vi "Main.vi"() -> ()   [LabVIEW 2013] (continued)
                n1844 = call "Msgbox - Message Handler.vi"("Short Description (When DB Not Available)"=w2943, "Description (When DB Not Available)"=w2949, "Post-Description"=w2946, "<.?....> Message Code"=w2944) -> ("MHandler Error"=w2950:errorcluster)  [unwired: 5 in, 2 out]
                n1845 = local write "MHandler"(w2950) -> ()
              }
            }
          }
          frame True {
            # "Must assume that ALL Captions are in Unicode IF IsUnicode is TRUE"
            # "Empty String in Mandatory Field"
            n1846 = call "Msgbox - Message Handler.vi"("Short Description (When DB Not Available)"="Part Details Incomplete" ("string"), "Description (When DB Not Available)"=" must be entered." ("message"), "Pre-Description"=w2960, "<.?....> Message Code"="<E 203>") -> ("MHandler Error"=w2964:errorcluster)  [unwired: 5 in, 2 out]
            n1847 = local write "MHandler"(w2964) -> ()
          }
        }
      }
      event "Part Details": Value Change {
        # "MCListbox Columns order# must match Item Details order#"
        # "USER Clicks on Part Details MCListBox (Also Called by Item No. Value Change}\nUpdate Edit Fields on Top"
        n1848 = event-data() -> ("CtlRef"=w3076:refnum<vi>, "NewVal"=w3070:i32)  [unwired: 1 in, 4 out]
        n1849 = disable-structure shown="Disabled" {
          frame Disabled {
            w3077 = ""
            # "Clear UI"
            n1850 = local write "[Remarks] +[ShortDescription] Debug"(w3077) -> ()
            n1851 = local write "[Remarks] +[ShortDescription]"(w3077) -> ()
          }
          frame Enabled {
          }
        }
        n1852 = property class="MCListbox (strict)"(reference=w3076) -> ("ColHdrString"=w3075:string[], "ItemNames"=w3069:string[][], "Value"=w3073:i32)  [unwired: 1 in, 2 out]
        n1853 = Index Array(array=w3069, index (row)=w3073) -> (element=w3074:string[])  [unwired: 1 in]
        n1854 = case shown="0, Default" w3073 {
          tunnel: w3075 -> [w3117 _]
          tunnel: w3074 -> [w3100 _]
          tunnel: [T30."Enabled" ("Disabled") T30."Disabled and Grayed Out" ("Disabled")] -> w3072
          tunnel: [w3101 T30."Disabled and Grayed Out" ("Disabled")] -> w3071
          tunnel: w3069 -> [_ _]
          frame 0, Default {
            # "Can look at Long Text"
            # "Don't Chnage User"
            # "Exisiting Parts Detail Record"
            n1855 = control-ref of="Item Details"() -> (w3116:refnum<vi>)
            n1856 = control-ref of="Channel Mapping"() -> (w3113:refnum<vi>)
            n1857 = control-ref of="Plot"() -> (w3110:refnum<vi>)
            n1858 = property class="Clust (strict)"(reference=w3116) -> ("Controls[]"=w3115:refnum<vi>[])  [unwired: 1 in, 2 out]
            n1859 = control-ref of="User"() -> ()  [unwired: 1 out]
            n1860 = property class="Clust (strict)"(reference=w3110) -> ("Controls[]"=w3109:refnum<vi>[])  [unwired: 1 in, 2 out]
            n1861 = property class="Clust (strict)"(reference=w3113) -> ("Controls[]"=w3112:refnum<vi>[])  [unwired: 1 in, 2 out]
            n1862 = control-ref of="Notes"() -> (w3114:refnum<vi>)
            n1863 = Build Array (concatenate)(w3115, w3114, w3112, w3109) -> (w3111:refnum<vi>[])
            n1864 = for {
              tunnel: w3111 -> [w3163] mode=indexing
              tunnel: w3117 -> [w3160]
              tunnel: w3100 -> [w3157]
              tunnel: [w3156] -> w3099
              tunnel: [w3156] -> w3107 mode=indexing
              n1865 = property class="Ctl"(reference=w3163) -> (reference out=w3161:refnum<vi>, "Label.Text"=w3159:string, "ClassName"=w3162:string)  [unwired: 1 in, 1 out]
              n1866 = Search 1D Array(1D array=w3160, element=w3159) -> (index of element=w3158:i32)  [unwired: 1 in]
              n1867 = case shown="0, Default" w3158 {
                selector: w3158 -> [w3165 _]
                tunnel: w3157 -> [w3169 _]
                tunnel: w3162 -> [w3168 _]
                tunnel: w3161 -> [w3166 _]
                tunnel: [w3164 _] -> w3156
                frame 0, Default {
                  n1868 = Index Array(array=w3169, index=w3165) -> (element=w3167:string)
                  n1869 = case shown="\"Boolean\"" w3168 {
                    tunnel: w3167 -> [w3172 w3176 w3179]
                    tunnel: w3166 -> [w3171 w3175 w3180]
                    tunnel: [w3170 w3174 w3177] -> w3164
                    frame "Digital" {
                      n1870 = Decimal String To Number(string=w3172) -> (number=w3173:i32)  [unwired: 2 in, 1 out]
                      n1871 = property class="Ctl"(reference=w3171, "Value"=w3173) -> (error out=w3170:errorcluster)  [unwired: 1 in, 1 out]
                    }
                    frame "ComboBox", "String", Default {
                      n1872 = property class="Ctl"(reference=w3175, "Value"=w3176) -> (error out=w3174:errorcluster)  [unwired: 1 in, 1 out]
                    }
                    frame "Boolean" {
                      n1873 = case shown="\"1\", \"T\", \"TRUE\", \"True\"" w3179 {
                        tunnel: [_ TRUE] -> w3178
                        frame "False", Default {
                        }
                        frame "1", "T", "TRUE", "True" {
                        }
                      }
                      n1874 = property class="Ctl"(reference=w3180, "Value"=w3178) -> (error out=w3177:errorcluster)  [unwired: 1 in, 1 out]
                    }
                  }
                }
                frame -1 {
                  # "Control Label not found in MCListBox ColHdrs"
                }
              }
            }
            n1875 = flat-sequence {
              tunnel: w3107 -> [_]
              frame #0 {
                # "<material>_<rev>_<description>.jpg"
                n1876 = control-ref of="Material"() -> (w3127:refnum<vi>)
                n1877 = control-ref of="Revision"() -> (w3126:refnum<vi>)
                n1878 = control-ref of="Material Description"() -> (w3125:refnum<vi>)
                n1879 = local read "DB - Master Data Load"() -> (w3121:bool)
                n1880 = property class="CmbBox"(reference=w3127) -> ("Value"=w3124:string)  [unwired: 1 in, 2 out]
                n1881 = property class="CmbBox"(reference=w3126) -> ("Value"=w3123:string)  [unwired: 1 in, 2 out]
                n1882 = property class="Str"(reference=w3125) -> ("Value"=w3122:string)  [unwired: 1 in, 2 out]
                n1883 = case shown="True" w3121 {
                  tunnel: w3124 -> [w3137 w3144]
                  tunnel: w3123 -> [w3136 w3143]
                  tunnel: w3122 -> [w3134 _]
                  tunnel: [w3128 w3141] -> w3120
                  tunnel: [w3130 w3140] -> w3119
                  tunnel: [w3129 _] -> w3118
                  frame False {
                    w3135 = "_"
                    # "No DB"
                    n1884 = Concatenate Strings(w3137, w3135, w3136, w3135, w3134, ".jpg" ("string")) -> (w3131:string)
                    n1885 = local read "MasterData\\JPG"() -> (w3132:path)
                    n1886 = Build Path(base path=w3132, name or relative path=w3131) -> (appended path=w3129:path)
                    n1887 = call <vilib>:"Read JPEG File.vi"("path to JPEG file"=w3129) -> ("error out"=w3128:errorcluster, "image data"=w3130:T40)  [unwired: 8 in, 1 out]
                  }
                  frame True {
                    # "Use DB"
                    n1888 = Bundle By Name(cluster=T12 {"Master Data Material"="", "Master Data Rev"="", "Master Data Material Description"="", "Inactive"=FALSE} ("Value"), "Master Data Material"=w3144, "Master Data Rev"=w3143) -> (w3145:T12)
                    n1889 = control-ref of="Material Buffer"() -> (w3147:refnum<vi>)
                    n1890 = local read "Logon"() -> (w3139:T21)
                    n1891 = property class="Clust (strict)"(reference=w3147, "Value"=w3145) -> (reference out=w3142:refnum<vi>)  [unwired: 1 in, 1 out]
                    n1892 = Unbundle By Name(w3139) -> ("LanguageID"=w3138:string)
                    n1893 = call "DB - [MasterData].[Material].vi"("DB - Master Data Material Enum"=DB_-_Master_Data_Material_Enum."SELECT [Description], [ImageFile]", "[LanguageId]"=w3138, "Clust Refnum"=w3142) -> ("image data"=w3140:T40, "SUMMARY"=w3141:errorcluster)  [unwired: 8 in, 3 out]
                  }
                }
                n1894 = case shown="No Error" w3120 {
                  tunnel: w3119 -> [w3150 _]
                  tunnel: w3118 -> [w3149 _]
                  frame No Error {
                    n1895 = control-ref of="Setup Thermocouple Location"() -> (w3154:refnum<vi>)
                    n1896 = Path To String(path=w3149) -> (string=w3152:string)
                    n1897 = call <vilib>:"Draw Flattened Pixmap.vi"("image data"=w3150, "picture"=picture data[5B]) -> ("new picture"=w3153:picture)  [unwired: 7 in]
                    n1898 = property class="Pict"(reference=w3154, "Desc"=w3152, "Value"=w3153) -> (error out=w3151:errorcluster)  [unwired: 1 in, 1 out]
                    n1899 = local write "Property Node Error"(w3151) -> ()
                  }
                  frame Error {
                  }
                }
              }
            }
            n1900 = property on="Material" class="CmbBox"(error in=w3099) -> (error out=w3106:errorcluster, "Value"=w3105:string)  [unwired: 1 in, 1 out]
            n1901 = local write "Property Node Error"(w3106) -> ()
            n1902 = Empty String/Path?(string/path=w3105) -> (empty?=w3104:bool)
            n1903 = Select(t=T30."Disabled and Grayed Out" ("Disabled"), s=w3104, f=T30."Enabled" ("Disabled")) -> (s? t:f=w3101:T30)
          }
          frame -1 {
            # "No Record"
          }
        }
        n1904 = flat-sequence {
          tunnel: w3070 -> [w3084]
          tunnel: w3069 -> [w3083]
          frame #0 {
            # "MClistBox Value Change EVENT\nThis Sequence Controls the ItemNo to show the Next Available Blank Record of the MCListBox\nThe other Suquence will be in the ItemNo Value Change EVENT which sets the MCListBox Value"
            n1905 = Array Size(array=w3083) -> (size(s)=w3082:i32[])
            n1906 = Index Array(array=w3082) -> (element=w3081:i32)  [unwired: 1 in]
            n1907 = case shown="-1" w3084 {
              selector: w3084 -> [w3090 _]
              tunnel: [w3094 w3097] -> w3080
              tunnel: w3081 -> [w3093 w3098]
              tunnel: [w3092 T30."Disabled and Grayed Out" ("Disabled")] -> w3079
              tunnel: [w3087 T30."Enabled" ("Disabled")] -> w3078
              frame 0, Default {
                # "Enable Add if new Record"
                # "Disable Delete if new Record"
                # "0 to LastValue+1"
                n1908 = Increment(x=w3090) -> (x+1=w3094:i32)
                n1909 = Greater?(x=w3094, y=w3093) -> (0:w3088:bool)
                n1910 = Select(t=T30."Enabled" ("Disabled"), s=w3088, f=T30."Disabled and Grayed Out" ("Disabled")) -> (s? t:f=w3087:T30)
                n1911 = Select(t=T30."Disabled and Grayed Out" ("Disabled"), s=w3088, f=T30."Enabled" ("Disabled")) -> (s? t:f=w3092:T30)
              }
              frame -1 {
                # "Nothing Selected\nGOTO next Record/Row"
                n1912 = Increment(x=w3098) -> (x+1=w3097:i32)
              }
            }
            n1913 = property on="Part Details Delete" class="Bool"("DisabledEnum"=w3079) -> ()  [unwired: 2 in, 2 out]
            n1914 = property on="Part Details Add" class="Bool (strict)"("DisabledEnum"=w3078) -> ()  [unwired: 2 in, 2 out]
            n1915 = local write "No."(w3080) -> ()
          }
        }
        n1916 = property on="SAPProduction Long Text" class="Bool"("DisabledEnum"=w3072) -> ()  [unwired: 2 in, 2 out]
        n1917 = property on="SAPMaterial Description (Long) Setup Tab" class="Bool"("DisabledEnum"=w3071) -> ()  [unwired: 2 in, 2 out]
      }
      event "No.": Value Change {
        # "Move the Cursor to point to the row in MCListbox"
        n1918 = event-data() -> ("NewVal"=w3186:i32)  [unwired: 1 in, 5 out]
        n1919 = property class="MCListbox (strict)"(reference=w3188) -> (reference out=w3184:refnum<vi>, "ItemNames"=w3185:string[][])  [unwired: 1 in, 1 out]
        n1920 = Number To Decimal String(number=w3186) -> (decimal integer string=w3190:string)  [unwired: 1 in]
        n1921 = flat-sequence {
          tunnel: w3186 -> [w3196]
          tunnel: w3185 -> [w3195]
          tunnel: w3184 -> [w3194]
          frame #0 {
            # "Upper Limit is ItemNames  #Rows + 1\nLower Limit is the smaller of 1 and #Rows"
            # "ItemNo Value Change EVENT\nThis Sequence Controls the MCListoBox Value to show\nThe other Sequence will be in the MCListBox Value Change EVENT which sets the ItemNo Value"
            n1922 = Array Size(array=w3195) -> (size(s)=w3202:i32[])
            n1923 = Index Array(array=w3202) -> (element=w3199:i32)  [unwired: 1 in]
            n1924 = Max & Min(x=w3199, y=1) -> (min(x,y)=w3200:i32)  [unwired: 1 out]
            n1925 = Increment(x=w3199) -> (x+1=w3197:i32)
            n1926 = In Range and Coerce(upper limit=w3197, x=w3196, lower limit=w3200) -> (coerced(x)=w3198:i32)  [unwired: 1 out]
            n1927 = Decrement(x=w3198) -> (x-1=w3193:i32)
            n1928 = disable-structure shown="Enabled" {
              disable-tunnel: w3194 -> [w3204 _]
              disable-tunnel: w3193 -> [w3203 _]
              frame Enabled {
                n1929 = property class="MCListbox (strict)"(reference=w3204, "Val(Sgnl)"=w3203) -> ()  [unwired: 1 in, 2 out]
              }
              frame Disabled {
              }
            }
          }
        }
        n1930 = Index Array(array=w3185, index (col)=0 ("disabled index (col)")) -> (element=w3191:string[])  [unwired: 1 in]
        n1931 = Search 1D Array(1D array=w3191, element=w3190) -> (index of element=w3189:i32)  [unwired: 1 in]
        n1932 = case shown="0, Default" w3189 {
          tunnel: [T30."Disabled and Grayed Out" ("Disabled") T30."Enabled" ("Disabled")] -> w3187
          frame 0, Default {
            # "No. Found in ItemNames"
          }
          frame -1 {
          }
        }
        n1933 = disable-structure shown="Enabled" {
          disable-tunnel: w3187 -> [_ w3206]
          frame Disabled {
            n1934 = property on="Part Details Add" class="Bool (strict)"() -> ("BoolText.Text"=w3205:string)  [unwired: 2 in, 2 out]
          }
          frame Enabled {
            n1935 = property on="Part Details Add" class="Bool (strict)"("DisabledEnum"=w3206) -> ()  [unwired: 2 in, 2 out]
          }
        }
      }
      event "Search [OrderNo] Toggle": Value Change {
        # "Get OrderNo Details from DB"
        n1936 = event-data() -> ()  [unwired: 1 in, 6 out]
        n1937 = property on="Order No." class="Str"() -> ("Value"=w3217:string)  [unwired: 2 in, 2 out]
        n1938 = call <vilib>:"Trim Whitespace.vi"("string"=w3217) -> ("trimmed string"=w3233:string)  [unwired: 1 in]
        n1939 = case shown="True" "DB - Setup Item (Part Details)" {
          tunnel: [_ w3238] -> w3215
          frame False {
          }
          frame True {
            # "Notes is not from SAP DB"
            # "To update Thermocouple Picture"
            # "Login\nItem Details\nWPS Details"
            n1940 = control-ref of="Item Details"() -> (w3245:refnum<vi>)
            n1941 = control-ref of="Notes"() -> ()  [unwired: 1 out]
            n1942 = Bundle By Name(cluster=T23 {"Item Details"=refnum, "WPS Details"=refnum, "WPS (Extra)"=refnum, "Rev (Extra) "=refnum, "FHS MCListbox"=refnum, "Additional WPS/Ref MCListBox"=refnum, "Notes"=refnum, "Part Details (MClistBox)"=refnum, "Result Output"=refnum} ("Refnums"), "Item Details"=w3245) -> (w3244:T23)
            n1943 = Build Array("SRTRS.Config.Mapping" ("DB.Schema.Table")) -> (w3243:string[])
            n1944 = call "DB - [Setup].[Item] (Part Details).vi"("DB - Setup Item Enum"=DB_-_Setup_Item_Enum."SELECT [Plant],[OrderNo]", "DB.Schema.Table Array"=w3243, "DB Refnums"=w3244) -> ("SUMMARY"=w3239:errorcluster)  [unwired: 7 in, 5 out]
            n1945 = local write "DB"(w3239) -> ()
            n1946 = property on="Revision" class="CmbBox"(error in=w3239, "Value"="") -> (error out=w3240:errorcluster)  [unwired: 1 in, 1 out]
            n1947 = property on="Revision Toggle" class="Str"(error in=w3240, "Val(Sgnl)"="Order No" ("Value (Signaling)")) -> (error out=w3238:errorcluster)  [unwired: 1 in, 1 out]
          }
        }
        n1948 = property on="Material" class="CmbBox"(error in=w3215) -> (error out=w3219:errorcluster, "Value"=w3226:string)  [unwired: 1 in, 1 out]
        n1949 = property on="NCR No." class="Str"(error in=w3215) -> (error out=w3210:errorcluster, "Value"=w3213:string)  [unwired: 1 in, 1 out]
        n1950 = call <vilib>:"Trim Whitespace.vi"("string"=w3213) -> ("trimmed string"=w3214:string)  [unwired: 1 in]
        n1951 = call <vilib>:"Trim Whitespace.vi"("string"=w3226) -> ("trimmed string"=w3227:string)  [unwired: 1 in]
        n1952 = Empty String/Path?(string/path=w3214) -> (empty?=w3212:bool)
        n1953 = Empty String/Path?(string/path=w3233) -> (empty?=w3220:bool)
        n1954 = Empty String/Path?(string/path=w3227) -> (empty?=w3222:bool)
        n1955 = Not(x=w3212) -> (.not. x?=w3211:bool)
        n1956 = Or(x=w3220, y=w3219) -> (x .or. y?=w3218:bool)
        n1957 = Or(x=w3222, y=w3219) -> (x .or. y?=w3221:bool)
        n1958 = property on="NCR Boolean" class="Bool (strict)"(error in=w3210, "Value"=w3211) -> (error out=w3209:errorcluster)  [unwired: 1 in, 1 out]
        n1959 = Select(t=T30."Disabled and Grayed Out" ("Disabled"), s=w3218, f=T30."Enabled" ("Disabled")) -> (s? t:f=w3231:T30)
        n1960 = Select(t=T30."Disabled and Grayed Out" ("Disabled"), s=w3221, f=T30."Enabled" ("Disabled")) -> (s? t:f=w3225:T30)
        n1961 = property on="SAPProduction Long Text" class="Bool"("DisabledEnum"=w3231) -> (error out=w3224:errorcluster)  [unwired: 2 in, 1 out]
        n1962 = property on="SAPMaterial Description (Long) Setup Tab" class="Bool"("DisabledEnum"=w3225) -> (error out=w3223:errorcluster)  [unwired: 2 in, 1 out]
        n1963 = Merge Errors(w3224, w3223, w3219, w3209) -> (w3216:errorcluster)
        n1964 = local write "Property Node Error"(w3216) -> ()
        n1965 = disable-structure shown="Disabled" {
          disable-tunnel: w3216 -> [w3235 _]
          frame Disabled {
            n1966 = flat-sequence {
              tunnel: w3235 -> [_]
              frame #0 {
                n1967 = property on="Oper. No." class="Str"("Key Focus"=TRUE) -> ()  [unwired: 2 in, 2 out]
                n1968 = Wait Until Next ms Multiple(millisecond multiple=u32 1000) -> ()  [unwired: 1 out]
              }
            }
          }
          frame Enabled {
          }
        }
      }
      event "Material.Master Data Rev": Value Change {
        # "From Either \nItem Details.Revision \nOR\nMaterial.Master Data Rev"
        n1969 = event-data() -> ("CtlRef"=w3250:refnum<vi>)  [unwired: 1 in, 5 out]
        n1970 = property class="CmbBox"(reference=w3250) -> ("Label.Text"=w3249:string)  [unwired: 1 in, 2 out]
        n1971 = case shown="\"Master Data Rev\"" w3249 {
          selector: w3249 -> [w3251 w3253]
          frame "Revision", Default {
            n1972 = property on="Revision Toggle" class="Str"("Val(Sgnl)"=w3251) -> ()  [unwired: 2 in, 2 out]
          }
          frame "Master Data Rev" {
            n1973 = local read "Master Data Ref Material"() -> (w3255:string)
            n1974 = String Length(string=w3255) -> (length=w3254:i32)
            n1975 = Equal To 0?(x=w3254) -> (x = 0?=w3252:bool)
            n1976 = case shown="True" w3252 {
              tunnel: w3253 -> [_ w3256]
              frame False {
              }
              frame True {
                n1977 = property on="Revision Toggle" class="Str"("Val(Sgnl)"=w3256) -> ()  [unwired: 2 in, 2 out]
              }
            }
          }
        }
      }
      event "No.": Key Down {
        n1978 = event-data() -> ("Char"=w3258:i16, "VKey"=w3259:T55)  [unwired: 1 in, 8 out]
        n1979 = case shown="\"Enter\", \"Return\"" w3259 {
          tunnel: w3258 -> [w3262 _]
          tunnel: [w3261 TRUE] -> w3257
          frame "ASCII", Default {
            n1980 = Equal?(x=w3262, y=i16 9) -> (x = y?=w3261:bool)
          }
          frame "Enter", "Return" {
          }
        }
        n1981 = case shown="True" w3257 {
          frame False {
          }
          frame True {
            n1982 = property on="Order No." class="Str"("Key Focus"=TRUE) -> ()  [unwired: 2 in, 2 out]
          }
        }
      }
      event Value Change {
        n1983 = event-data() -> ("NewVal"=w3267:string)  [unwired: 1 in, 5 out]
        n1984 = Empty String/Path?(string/path=w3267) -> (empty?=w3266:bool)
        n1985 = Not(x=w3266) -> (.not. x?=w3265:bool)
        n1986 = property on="NCR Boolean" class="Bool (strict)"("Value"=w3265) -> ()  [unwired: 2 in, 2 out]
      }
      event "Channel Mapping", "Channel Mapping.TC1", "Channel Mapping.TC2", "Channel Mapping.TC3", "Channel Mapping.TC4", "Channel Mapping.TC5", "Channel Mapping.TC6": Key Down? {
        n1987 = event-data() -> ("CtlRef"=w3271:refnum<vi>, "Char"=w3269:i16, "VKey"=w3268:T55)  [unwired: 1 in, 7 out]
        n1988 = case shown="\"Enter\", \"Return\"" w3268 {
          selector: w3268 -> [w3288 _]
          tunnel: [w3289 w3291] -> w3274
          tunnel: w3269 -> [w3289 _]
          tunnel: [w3288 eventvkey."ASCII" ("VKey")] -> w3273
          frame "ASCII", Default {
            # "Key in TAB"
          }
          frame "Enter", "Return" {
            w3291 = i16 9  # TAB
          }
        }
        n1989 = case "Only NUMBERS, BackSpace, TAB and (Up, Down, Right, Left, Delete)" shown="0, Default" w3269 {
          tunnel: [w3292 w3296] -> w3272
          tunnel: w3268 -> [w3293 _]
          frame 0, Default {
            # "Exception"
            n1990 = case shown="\"Enter\", \"Return\", \"Up\"..\"Right\", \"Delete\"" w3293 {
              tunnel: [w3294 w3295] -> w3292
              frame Default {
                w3294 = TRUE  # Discard
              }
              frame "Enter", "Return", "Up".."Right", "Delete" {
                w3295 = FALSE  # Do Not Discard
                # "Up, Down, Left, Right, Delete, Enter Return"
              }
            }
          }
          frame 8, 9, 48..57 {
            w3296 = FALSE  # Do not discard
            # "Char\n48-57  Numbers\n58        . (decimal Point)\n46        : (colon)\n8          Backspace\n9          TAB"
            # "Numbers and Backspace"
          }
        }
        n1991 = property class="Ctl"(reference=w3271) -> ("Label.Text"=w3270:string)  [unwired: 1 in, 2 out]
        n1992 = case shown="False" w3272 {
          tunnel: w3270 -> [w3277 _]
          tunnel: w3269 -> [w3276 _]
          tunnel: w3268 -> [w3275 _]
          frame False {
            # "Set TRUE to Plot0# as soon as Key Down? for TC#\nSet FALSE will be done at Item Details Value Change"
            n1993 = case shown="0, Default" w3276 {
              tunnel: w3277 -> [w3279 _]
              tunnel: w3275 -> [w3278 _]
              frame 0, Default {
                n1994 = case shown="\"ASCII\"" w3278 {
                  tunnel: w3279 -> [_ w3281]
                  frame Default {
                    # "Enter, Return"
                  }
                  frame "ASCII" {
                    n1995 = Search 1D Array(1D array=string[] ["TC1", "TC2", "TC3", "TC4", "TC5", "TC6"], element=w3281) -> (index of element=w3280:i32)  [unwired: 1 in]
                    n1996 = property on="Plot" class="Clust (strict)"() -> ("Value"=w3287:T4)  [unwired: 2 in, 2 out]
                    n1997 = Cluster To Array(cluster=w3287) -> (array=w3286:bool[])
                    n1998 = Replace Array Subset(array=w3286, new element=TRUE, index=w3280) -> (w3284:bool[])
                    n1999 = Array To Cluster "Size=6"(array=w3284) -> (cluster=w3283:T70)
                    n2000 = property on="Plot" class="Clust (strict)"("Value"=w3283) -> ()  [unwired: 2 in, 2 out]
                  }
                }
              }
              frame 8, 9 {
                # "Ignore Backspace. User may be deleting a blank entry.\nIgnore TAB"
              }
            }
          }
          frame True {
          }
        }
        n2001 = event-data("Discard?"=w3272, "Char"=w3274, "VKey"=w3273) -> ()  [unwired: 1 in, 1 out]
      }
      event Key Down {
        # "Move Cursor to a different field when Return, Enter or TAB is pressed"
        n2002 = event-data() -> ("CtlRef"=w3297:refnum<vi>, "Char"=w3300:i16, "VKey"=w3299:T55)  [unwired: 1 in, 7 out]
        n2003 = case shown="\"ASCII\", Default" w3299 {
          tunnel: w3300 -> [w3325 _]
          tunnel: [w3324 TRUE] -> w3298
          frame "ASCII", Default {
            w3326 = i16 9  # TAB
            n2004 = Equal?(x=w3325, y=w3326) -> (x = y?=w3324:bool)
          }
          frame "Enter", "Return" {
          }
        }
        n2005 = case shown="True" w3298 {
          tunnel: w3297 -> [_ w3305]
          frame False {
          }
          frame True {
            # "SKIP NCR Boolean\nSerial No. is the last entry"
            n2006 = property class="Ctl"(reference=w3305) -> (reference out=w3307:refnum<vi>, "Label.Text"=w3306:string)  [unwired: 1 in, 1 out]
            n2007 = control-ref of="Item Details"() -> (w3309:refnum<vi>)
            n2008 = property class="Clust (strict)"(reference=w3309) -> ("Controls[]"=w3302:refnum<vi>[])  [unwired: 1 in, 2 out]
            n2009 = Search 1D Array(1D array=w3302, element=w3305) -> (index of element=w3308:i32)  [unwired: 1 in]
            n2010 = Increment(x=w3308) -> (x+1=w3301:i32)
            n2011 = case shown="\"NCR No.\"" w3306 {
              tunnel: w3307 -> [_ _ _ _]
              tunnel: [w3312 w3315 w3320 w3323] -> w3303
              tunnel: w3302 -> [w3314 w3317 w3322 _]
              tunnel: w3301 -> [w3313 w3316 w3321 _]
              frame "NCR No." {
                # "SKIP NCR Boolean"
                n2012 = Add(x=1, y=w3313) -> (x+y=w3311:i32)
                n2013 = Index Array(array=w3314, index=w3311) -> (element=w3312:refnum<vi>)
              }
              frame "Order No." {
                n2014 = property on="Search [OrderNo] Toggle" class="Bool (strict)"() -> ("Value"=w3319:bool)  [unwired: 2 in, 2 out]
                n2015 = Index Array(array=w3317, index=w3316) -> (element=w3315:refnum<vi>)
                n2016 = Not(x=w3319) -> (.not. x?=w3318:bool)
                n2017 = property on="Search [OrderNo] Toggle" class="Bool (strict)"("Val(Sgnl)"=w3318) -> ()  [unwired: 2 in, 2 out]
              }
              frame Default {
                # "TAB to next"
                n2018 = Index Array(array=w3322, index=w3321) -> (element=w3320:refnum<vi>)
              }
              frame "Serial No." {
                # "Last"
                n2019 = control-ref of="TC1"() -> (w3323:refnum<vi>)
              }
            }
            n2020 = property class="Ctl"(reference=w3303, "Key Focus"=TRUE) -> ()  [unwired: 1 in, 2 out]
          }
        }
      }
      event Key Down? {
        n2021 = event-data() -> ("VKey"=w3328:T55)  [unwired: 1 in, 9 out]
        n2022 = case shown="\"Down\"" w3328 {
          frame "ASCII", Default {
          }
          frame "Down" {
            # "<material>_<rev>_<description>.jpg"
            # "<wps/ref>_<rev>.wps"
            # "If user clicks on DOWN arrow key"
            n2023 = local read "MasterData\\JPG"() -> (w3330:path)
            n2024 = control-ref of="Material"() -> (w3329:refnum<vi>)
            n2025 = List Folder(path=w3330, pattern="*.jpg") -> (filenames=w3331:string[])  [unwired: 2 in, 3 out]
            n2026 = call "String - Extract Unique Headers_.vi"("Array In"=w3331) -> ("Array Out"=w3332:string[])  [unwired: 10 in]
            n2027 = local write "Temp Array"(w3331) -> ()
            n2028 = property class="CmbBox"(reference=w3329, "Strings[]"=w3332) -> ()  [unwired: 1 in, 2 out]
          }
        }
        n2029 = event-data() -> ()  [unwired: 2 in, 1 out]
      }
      event "Channel Mapping", "Notes", "Plot": Value Change {
        # "USER Changed Item Details"
        # "To cater for Mouse Click outside of Editing Fields"
        n2030 = event-data() -> ()  [unwired: 1 in, 6 out]
        n2031 = property class="MCListbox (strict)"(reference=w3336) -> ("Value"=w3335:i32)  [unwired: 1 in, 2 out]
        n2032 = Greater Or Equal To 0?(x=w3335) -> (x >= 0?=w3334:bool)
        n2033 = case shown="True" w3334 {
          tunnel: w3336 -> [_ w3348]
          frame False {
            # "User NOT editiing current item from MClistBox"
          }
          frame True {
            # "No. is already in the ItemNames"
            # "User editing current Item in MCListbox"
            n2034 = property class="MCListbox (strict)"(reference=w3348) -> ("ItemNames"=w3347:string[][])  [unwired: 1 in, 2 out]
            n2035 = local read "No."() -> (w3346:i32)
            n2036 = local read "Setup Edit"() -> (w3341:bool)
            n2037 = disable-structure shown="Disabled" {
              frame Disabled {
                n2038 = property on="Part Details Add" class="Bool (strict)" props=["DisabledEnum"]() -> ()  [unwired: 2 in, 3 out]
              }
              frame Enabled {
              }
            }
            n2039 = Index Array(array=w3347, index (col)=0 ("disabled index (col)")) -> (element=w3344:string[])  [unwired: 1 in]
            n2040 = Number To Decimal String(number=w3346) -> (decimal integer string=w3345:string)  [unwired: 1 in]
            n2041 = property on="Channel Mapping" class="Clust (strict)"() -> ("Value"=w3338:T2)  [unwired: 2 in, 2 out]
            n2042 = Search 1D Array(1D array=w3344, element=w3345) -> (index of element=w3342:i32)  [unwired: 1 in]
            n2043 = Cluster To Array(cluster=w3338) -> (array=w3337:string[])
            n2044 = Greater Or Equal To 0?(x=w3342) -> (x >= 0?=w3340:bool)
            n2045 = And(x=w3341, y=w3340) -> (x .and. y?=w3339:bool)
            n2046 = for {
              tunnel: w3337 -> [w3352] mode=indexing
              i -> [w3349]
              n2047 = call <vilib>:"Trim Whitespace.vi"("string"=w3352) -> ("trimmed string"=w3351:string)  [unwired: 1 in]
              n2048 = Empty String/Path?(string/path=w3351) -> (empty?=w3350:bool)
              n2049 = case shown="True" w3350 {
                tunnel: w3349 -> [_ w3355]
                frame False {
                }
                frame True {
                  # "Empty TC#\nUncheck Plot0#"
                  n2050 = property on="Plot" class="Clust (strict)"() -> ("Value"=w3358:T4)  [unwired: 2 in, 2 out]
                  n2051 = Cluster To Array(cluster=w3358) -> (array=w3357:bool[])
                  n2052 = Replace Array Subset(array=w3357, new element=FALSE, index=w3355) -> (w3354:bool[])
                  n2053 = Array To Cluster(array=w3354) -> (cluster=w3353:T70)
                  n2054 = property on="Plot" class="Clust (strict)"("Value"=w3353) -> ()  [unwired: 2 in, 2 out]
                }
              }
            }
            n2055 = case shown="True" w3339 {
              frame False {
              }
              frame True {
                # "Edit Mode"
                n2056 = property on="Part Details Add" class="Bool (strict)"("Val(Sgnl)"=TRUE) -> ()  [unwired: 2 in, 2 out]
              }
            }
          }
        }
      }
      event "Channel Mapping.TC1", "Channel Mapping.TC2", "Channel Mapping.TC3", "Channel Mapping.TC4", "Channel Mapping.TC5", "Channel Mapping.TC6", "Plot.TC01Plot", "Plot.TC02Plot", "Plot.TC03Plot", "Plot.TC04Plot", "Plot.TC05Plot", "Plot.TC06Plot": Key Down {
        # "Move Cursor to a different field when Return, Enter or TAB is pressed"
        n2057 = event-data() -> ("CtlRef"=w3361:refnum<vi>, "Char"=w3363:i16, "VKey"=w3362:T55)  [unwired: 1 in, 7 out]
        n2058 = case shown="\"ASCII\", Default" w3362 {
          tunnel: w3363 -> [w3400 _]
          tunnel: [w3399 TRUE] -> w3360
          frame "ASCII", Default {
            n2059 = Equal?(x=w3400, y=i16 9) -> (x = y?=w3399:bool)
          }
          frame "Enter", "Return" {
          }
        }
        n2060 = case shown="True" w3360 {
          tunnel: w3361 -> [_ w3372]
          frame False {
          }
          frame True {
            n2061 = disable-structure shown="Enabled" {
              frame Disabled {
                n2062 = property on="Part Details Add" class="Bool (strict)"() -> ("BoolText.Text"=w3390:string)  [unwired: 2 in, 2 out]
                n2063 = case shown="\"Edit\"" w3390 {
                  frame "False", Default {
                  }
                  frame "Edit" {
                    n2064 = property on="Part Details Add" class="Bool (strict)"("Val(Sgnl)"=TRUE) -> ()  [unwired: 2 in, 2 out]
                  }
                }
              }
              frame Enabled {
                n2065 = property on="Part Details Add" class="Bool (strict)"() -> ("DisabledEnum"=w3392:T30)  [unwired: 2 in, 2 out]
                n2066 = case shown="\"Disabled and Grayed Out\"" w3392 {
                  frame "Enabled", Default {
                  }
                  frame "Disabled and Grayed Out" {
                    # "Edit Mode"
                    n2067 = property on="Part Details Add" class="Bool (strict)"("Val(Sgnl)"=TRUE) -> ()  [unwired: 2 in, 2 out]
                  }
                }
              }
            }
            n2068 = control-ref of="Plot"() -> (w3370:refnum<vi>)
            n2069 = control-ref of="Channel Mapping"() -> (w3375:refnum<vi>)
            n2070 = property class="Clust (strict)"(reference=w3370) -> ("Controls[]"=w3365:refnum<vi>[])  [unwired: 1 in, 2 out]
            n2071 = property class="Clust (strict)"(reference=w3375) -> ("Controls[]"=w3369:refnum<vi>[])  [unwired: 1 in, 2 out]
            n2072 = Build Array (concatenate)(w3369, w3365) -> (w3368:refnum<vi>[])
            n2073 = Search 1D Array(1D array=w3368, element=w3372) -> (index of element=w3364:i32)  [unwired: 1 in]
            n2074 = property class="Ctl"(reference=w3372) -> (reference out=w3366:refnum<vi>, "Label.Text"=w3367:string)  [unwired: 1 in, 1 out]
            n2075 = Increment(x=w3364) -> (x+1=w3371:i32)
            n2076 = disable-structure shown="Disabled" {
              disable-tunnel: w3367 -> [w3379 _]
              disable-tunnel: w3366 -> [w3378 _]
              disable-tunnel: w3365 -> [w3377 _]
              disable-tunnel: w3364 -> [w3376 _]
              frame Disabled {
                n2077 = case shown="\"TC1\", \"TC2\", \"TC3\", \"TC4\", \"TC5\", \"TC6\"" w3379 {
                  tunnel: w3378 -> [_ w3385]
                  tunnel: w3377 -> [_ w3384]
                  tunnel: w3376 -> [_ w3383]
                  frame "False", Default {
                  }
                  frame "TC1", "TC2", "TC3", "TC4", "TC5", "TC6" {
                    w3389 = refnum<vi> refnum  # String
                    n2078 = To More Specific Class(target class=w3389, reference=w3385) -> (specific class reference=w3388:refnum<vi>)  [unwired: 1 in, 1 out]
                    n2079 = property class="Str"(reference=w3388) -> ("Value"=w3387:string)  [unwired: 1 in, 2 out]
                    n2080 = call <vilib>:"Trim Whitespace.vi"("string"=w3387) -> ("trimmed string"=w3386:string)  [unwired: 1 in]
                    n2081 = Empty String/Path?(string/path=w3386) -> (empty?=w3381:bool)
                    n2082 = Index Array(array=w3384, index=w3383) -> (element=w3382:refnum<vi>)
                    n2083 = Not(x=w3381) -> (.not. x?=w3380:bool)
                    n2084 = property class="Ctl"(reference=w3382, "Value"=w3380) -> ()  [unwired: 1 in, 2 out]
                  }
                }
              }
              frame Enabled {
              }
            }
            n2085 = case shown="\"TC6\"" w3367 {
              tunnel: [w3394 w3395 w3396] -> w3373
              tunnel: w3366 -> [_ _ _]
              tunnel: w3368 -> [_ _ w3398]
              tunnel: w3371 -> [_ _ w3397]
              frame "TC6" {
                # "Last"
                n2086 = control-ref of="TC01Plot"() -> (w3394:refnum<vi>)
              }
              frame "TC06Plot" {
                n2087 = control-ref of="Notes"() -> (w3395:refnum<vi>)
              }
              frame Default {
                n2088 = Index Array(array=w3398, index=w3397) -> (element=w3396:refnum<vi>)
              }
            }
            n2089 = property class="Ctl"(reference=w3373, "Key Focus"=TRUE) -> ()  [unwired: 1 in, 2 out]
          }
        }
      }
      event "Notes", "User": Key Down {
        # "Move Cursor to a different field when Return, Enter or TAB is pressed"
        n2090 = event-data() -> ("CtlRef"=w3404:refnum<vi>, "Char"=w3406:i16, "VKey"=w3405:T55)  [unwired: 1 in, 7 out]
        n2091 = case shown="\"Enter\", \"Return\"" w3405 {
          tunnel: w3406 -> [w3413 _]
          tunnel: [w3412 TRUE] -> w3403
          frame "ASCII", Default {
            n2092 = Equal?(x=w3413, y=i16 9) -> (x = y?=w3412:bool)
          }
          frame "Enter", "Return" {
          }
        }
        n2093 = case shown="True" w3403 {
          tunnel: w3404 -> [_ _]
          frame False {
          }
          frame True {
            # "If in Edit Mode, do a Part Details Add"
            n2094 = disable-structure shown="Disabled" {
              frame Disabled {
                n2095 = property on="Part Details Add" class="Bool (strict)"() -> ("BoolText.Text"=w3407:string)  [unwired: 2 in, 2 out]
                n2096 = case shown="\"Edit\"" w3407 {
                  frame "False", Default {
                    n2097 = property on="Part Details Add" class="Bool (strict)"("Key Focus"=TRUE) -> ()  [unwired: 2 in, 2 out]
                  }
                  frame "Edit" {
                    n2098 = property on="Part Details Add" class="Bool (strict)"("Val(Sgnl)"=TRUE) -> ()  [unwired: 2 in, 2 out]
                  }
                }
              }
              frame Enabled {
                n2099 = property on="Part Details Add" class="Bool (strict)"() -> ("DisabledEnum"=w3410:T30)  [unwired: 2 in, 2 out]
                n2100 = case shown="\"Disabled and Grayed Out\"" w3410 {
                  frame "Enabled", Default {
                  }
                  frame "Disabled and Grayed Out" {
                    n2101 = property on="Part Details Add" class="Bool (strict)"("Val(Sgnl)"=TRUE) -> ()  [unwired: 2 in, 2 out]
                  }
                }
              }
            }
          }
        }
      }
      event "------------------------------------        Master Data       -----------------------------------": Value Change {
        n2102 = event-data() -> ()  [unwired: 1 in, 6 out]
      }
      event "Master Data New": Value Change {
        w3427 = 4 ("dimension size")
        # "MasterData WPS"
        n2103 = event-data() -> ()  [unwired: 1 in, 6 out]
        n2104 = call "Msgbox - Message Handler.vi"("Short Description (When DB Not Available)"="Create New WPS", "Description (When DB Not Available)"="All unsaved data will be lost. Do you want to proceed?", "<.?....> Message Code"="<W 521>") -> ("MHandler Error"=→"MHandler":errorcluster, "OK Out"=w3419:bool)  [unwired: 6 in, 1 out]
        n2105 = control-ref of="MCListBox FHS Master Data"() -> (w3425:refnum<vi>)
        n2106 = Initialize Array("", w3427) -> (w3430:string[])
        n2107 = Build Array(w3430) -> (w3429:string[][])
        n2108 = case shown="True" w3419 {
          frame False {
          }
          frame True {
            w3432 = ""
            # "Temperature Units is from ini file,\nso default value may not be correct"
            n2109 = global read "Global SRTRS.vi" "Temperature Units"() -> (w3431:string)
            n2110 = control-ref of="WPS Details Master Data"() -> (w3437:refnum<vi>)
            n2111 = property class="Clust (strict)"(reference=w3437) -> (reference out=w3436:refnum<vi>, "Value"=w3435:T13)  [unwired: 1 in, 1 out]
            n2112 = Bundle By Name(cluster=w3435, "Master Data WPS/Ref"=w3432, "Master Data Rev"=w3432, "Master Data Hold Temperature"=w3432, "Master Data Temperature Units"=w3431, "Master Data Hold Time (HH:MM)"=w3432, "Inactive"=FALSE) -> (w3434:T13)
            n2113 = property class="Clust (strict)"(reference=w3436, "Value"=w3434) -> ()  [unwired: 1 in, 2 out]
          }
        }
        n2114 = property on="Property Node" class="MCListbox (strict)"(reference=w3425, "ItemNames"=w3429, "NumCols"=w3427) -> (reference out=w3426:refnum<vi>)  [unwired: 1 in, 1 out]
        n2115 = local read "CellBG Unused Cells"() -> (w3423:u32)
        n2116 = local read "CellBG New Cells"() -> (w3422:u32)
        n2117 = property on="Master Data Rev" class="CmbBox (strict)"("Strings[]"=string[] [] ("Strings []")) -> ()  [unwired: 2 in, 2 out]
        n2118 = call "MCListbox Refresh.vi"("Which Cells"=T46."Exisiting and Blank Cells", "color of New Cells"=w3422, "color of Blank cells"=w3423, "MulticolumnListbox in"=w3426) -> ()  [unwired: 6 in, 2 out]
      }
      event "Master Data Save", "Master Data Delete": Value Change {
        # "{Save WPS} and {Delete} (Legacy)"
        n2119 = event-data() -> ("CtlRef"=w3447:refnum<vi>)  [unwired: 1 in, 5 out]
        n2120 = property class="Bool"(reference=w3447) -> ("Label.Text"=w3446:string)  [unwired: 1 in, 2 out]
        n2121 = Unbundle By Name("WPS Details Master Data") -> ("Master Data WPS/Ref"=w3445:T5, "Master Data Rev"=w3444:T5, "Master Data Hold Temperature"=w3443:string, "Master Data Hold Time (HH:MM)"=w3442:string)
        n2122 = Empty String/Path?(string/path=w3442) -> (empty?=w3439:bool)
        n2123 = Empty String/Path?(string/path=w3443) -> (empty?=w3440:bool)
        n2124 = Empty String/Path?(string/path=w3445) -> (empty?=w3441:bool)
        n2125 = Compound Arithmetic op=OR(w3441, w3440, w3439) -> (w3438:bool)
        n2126 = case shown="True" w3438 {
          tunnel: w3446 -> [w3453 w3633]
          tunnel: w3445 -> [w3452 _]
          tunnel: w3444 -> [w3451 _]
          tunnel: [w3449 FALSE ("Skip Final Prompt")] -> _
          frame False {
            # "Complete Fields in Header"
            n2127 = local read "MasterData\\WPS"() -> (w3454:path)
            n2128 = Concatenate Strings(w3452, "_" ("string"), w3451, ".wps" ("string")) -> (w3450:string)
            n2129 = Build Path(base path=w3454, name or relative path=w3450) -> (appended path=w3457:path)
            n2130 = case shown="\"Master Data Save\"" w3453 {
              tunnel: w3457 -> [w3463 w3535]
              tunnel: w3450 -> [w3461 _]
              tunnel: [w3460 TRUE ("Skip Final Prompt")] -> w3449
              frame "Master Data Delete", Default {
                # "Only NO DB here"
                # "Master Data Delete. Same as Master Data New - need to clear everything"
                n2131 = call <vilib>:"Check if File or Folder Exists.vi"("path"=w3463) -> ("file or folder exists?"=w3462:bool)  [unwired: 8 in, 2 out]
                n2132 = case shown="True" w3462 {
                  tunnel: w3463 -> [w3466 w3480]
                  tunnel: w3461 -> [_ w3478]
                  tunnel: [w3465 w3475] -> w3458
                  tunnel: [TRUE ("Skip Final Prompt") w3474] -> w3460
                  frame False {
                    w3471 = "\"" ("string")
                    # "File to Delete not found"
                    n2133 = Path To String(path=w3466) -> (string=w3472:string)
                    n2134 = Concatenate Strings("[Delete WPS]" ("string"), " Not OK." ("string"), "\n") -> (w3468:string)
                    n2135 = Concatenate Strings(w3468, w3471, w3472, w3471, " Not Found. " ("string")) -> (w3465:string)
                  }
                  frame True {
                    # "File to be deleted is found"
                    n2136 = Concatenate Strings("Confirm Delete " ("string"), w3478) -> (w3477:string)
                    n2137 = Two Button Dialog(message=w3477) -> (T button?=w3476:bool)  [unwired: 2 in]
                    n2138 = case shown="True" w3476 {
                      tunnel: w3480 -> [_ w3505]
                      tunnel: [w3484 w3490] -> w3475
                      tunnel: [w3483 TRUE ("Skip Final Prompt")] -> w3474
                      frame False {
                        w3483 = FALSE  # Skip Final Prompt
                        # "User Cancels Delete"
                        n2139 = Concatenate Strings("{Delete WPS}" ("string"), " Cancelled.", "\n") -> (w3484:string)
                      }
                      frame True {
                        w3501 = 3 ("dimension size")
                        # "Temperature Units is from ini file,\nso default value may not be correct"
                        # "User OKs delete"
                        n2140 = Delete(path (use dialog)=w3505) -> (deleted path=w3491:path, error out=w3492:errorcluster)  [unwired: 4 in, 1 out]
                        n2141 = control-ref of="MCListBox FHS Master Data"() -> (w3499:refnum<vi>)
                        n2142 = control-ref of="WPS Details Master Data"() -> (w3498:refnum<vi>)
                        n2143 = property on="Master Data Temperature Units" class="Str"() -> (error out=w3497:errorcluster, "Value"=w3495:string)  [unwired: 2 in, 1 out]
                        n2144 = Initialize Array("", w3501) -> (w3504:string[])
                        n2145 = Build Array(w3504) -> (w3503:string[][])
                        n2146 = invoke class="Clust (strict)" method="Reinit To Default"(reference=w3498, error in=w3497) -> (error out=w3496:errorcluster)  [unwired: 1 in, 2 out]
                        n2147 = property on="Property Node" class="MCListbox (strict)"(reference=w3499, "ItemNames"=w3503, "NumCols"=w3501) -> (reference out=w3500:refnum<vi>)  [unwired: 1 in, 1 out]
                        n2148 = local read "CellBG Unused Cells"() -> (w3488:u32)
                        n2149 = local read "CellBG New Cells"() -> (w3487:u32)
                        n2150 = property on="Master Data Rev" class="CmbBox (strict)"("Strings[]"=string[] [] ("Strings []")) -> ()  [unwired: 2 in, 2 out]
                        n2151 = property on="Master Data Temperature Units" class="Str"(error in=w3496, "Value"=w3495) -> ()  [unwired: 1 in, 2 out]
                        n2152 = call "MCListbox Refresh.vi"("Which Cells"=T46."Exisiting and Blank Cells", "color of New Cells"=w3487, "color of Blank cells"=w3488, "MulticolumnListbox in"=w3500) -> ()  [unwired: 6 in, 2 out]
                        n2153 = case shown="No Error" w3492 {
                          tunnel: w3491 -> [w3514 _]
                          tunnel: [w3510 w3517] -> w3490
                          tunnel: "{Delete WPS}" ("string") -> [w3508 w3516]
                          frame No Error {
                            w3512 = "\"" ("string")
                            # "File Delete OK"
                            n2154 = Path To String(path=w3514) -> (string=w3513:string)
                            n2155 = Concatenate Strings(w3508, " OK." ("string"), "\n") -> (w3507:string)
                            n2156 = Concatenate Strings(w3507, w3512, w3513, w3512, " deleted. " ("string")) -> (w3510:string)
                          }
                          frame Error {
                            # "File Delete Not OK"
                            n2157 = Concatenate Strings(w3516, " Not OK.", "\n") -> (w3517:string)
                          }
                        }
                      }
                    }
                  }
                }
                n2158 = call "Queue - EnQueue to MessageQ.vi"("<NoD> Don't Display to UI"=TRUE, "Message"=w3458) -> ()  [unwired: 9 in, 1 out]
              }
              frame "Master Data Save" {
                w3519 = TRUE ("Check and Add Empty Row if Needed")
                # "This part needed in case user click on SAVE bypassing the checks\ndone on MCListbox"
                n2159 = control-ref of="MCListBox FHS Master Data"() -> (w3522:refnum<vi>)
                n2160 = property class="MCListbox (strict)"(reference=w3522) -> (reference out=w3532:refnum<vi>, "ItemNames"=w3533:string[][])  [unwired: 1 in, 1 out]
                n2161 = call "String - Sort Array.vi"("Force Running Numbers"=w3519, "Check and Add Empty Row if Needed"=w3519, "2D Array in"=w3533) -> ("2D Array out"=w3520:string[][])  [unwired: 6 in, 2 out]
                n2162 = property class="MCListbox (strict)"(reference=w3532, "ItemNames"=w3520) -> (reference out=w3526:refnum<vi>)  [unwired: 1 in, 1 out]
                n2163 = call "String - Check Empty Cells.vi"("ItemNames"=w3520) -> ("Rows > 0"=w3521:bool, "Location of Empty Cell (R,C)"=w3523:i32[][], "Empty Cell(s)"=w3524:bool)  [unwired: 8 in]
                n2164 = call "MCListbox Event - Key Down.vi"("VKey"=eventvkey."Enter", "CtlRef"=w3526) -> ("Error Out"=w3525:errorcluster)  [unwired: 8 in, 1 out]
                n2165 = local read "CellBG Unused Cells"() -> (w3528:u32)
                n2166 = local read "CellBG New Cells"() -> (w3529:u32)
                n2167 = call "MCListbox Refresh.vi"("Which Cells"=T46."Exisiting and Blank Cells", "Error In"=w3525, "color of New Cells"=w3529, "color of Blank cells"=w3528, "MulticolumnListbox in"=w3526) -> ("MulticolumnListbox out"=w3527:refnum<vi>)  [unwired: 5 in, 1 out]
                n2168 = case shown="False" w3524 {
                  tunnel: w3535 -> [w3550 _]
                  tunnel: w3527 -> [_ _]
                  tunnel: w3523 -> [_ w3613]
                  tunnel: w3522 -> [w3543 w3614]
                  tunnel: w3521 -> [_ w3603]
                  tunnel: w3520 -> [w3544 _]
                  frame False {
                    # "Otherwise the Last Row will be\nin EditPosition Mode"
                    # "No Empty Cells"
                    n2169 = control-ref of="WPS Details Master Data"() -> (w3548:refnum<vi>)
                    n2170 = property class="Clust (strict)"(reference=w3548) -> ("Value"=w3547:T13)  [unwired: 1 in, 2 out]
                    n2171 = property class="MCListbox (strict)"(reference=w3543, "Value"=-1, "Key Focus"=FALSE) -> ()  [unwired: 1 in, 2 out]
                    n2172 = Unbundle By Name(w3547) -> ("Master Data Hold Temperature"=w3549:string, "Master Data Hold Time (HH:MM)"=w3546:string)
                    n2173 = call "String - Check Hold Parameters.vi"("Master Data Hold Time (HH:MM)"=w3546, "Master Data Hold Temperature"=w3549, "2D Array in"=w3544) -> ("Found"=w3545:bool)  [unwired: 6 in, 2 out]
                    n2174 = case shown="True" w3545 {
                      tunnel: w3550 -> [_ w3563]
                      tunnel: w3543 -> [_ w3566]
                      tunnel: w3548 -> [_ w3560]
                      tunnel: ["Hold. Temperature  or Hold Time does not match in Heating Sequence. " ("string") w3564] -> w3541
                      tunnel: [_ w3554] -> w3540
                      tunnel: ["<E 209>" ("string") w3558] -> w3539
                      tunnel: ["WPS Error." ("string") w3557] -> w3538
                      frame False {
                        # "Matching Hold Temp and Time NOT FOUND"
                      }
                      frame True {
                        # "Matching Hold Temp and Time FOUND"
                        n2175 = case shown="True" "DB - Master Data Save" {
                          tunnel: [w3567 w3583] -> w3561
                          tunnel: w3563 -> [w3575 _]
                          tunnel: w3566 -> [w3574 w3584]
                          tunnel: w3560 -> [w3573 w3582]
                          tunnel: w3563 -> [w3569 _]
                          tunnel: [w3568 _] -> w3562
                          frame False {
                            w3571 = "\"" ("string")
                            # "Use File"
                            n2176 = call <vilib>:"Open Config Data.vi"("configuration file path"=w3575) -> ("error out"=w3580:errorcluster, "refnum"=w3581:T59)  [unwired: 8 in, 1 out]
                            n2177 = call "Key - Cluster Write.vi"("error in (no error)"=w3580, "Cluster Ref in"=w3573, "Refnum in"=w3581) -> ("error out"=w3578:errorcluster, "Refnum out"=w3579:T59)  [unwired: 7 in]
                            n2178 = call "Key - MCListbox Write.vi"("error in (no error)"=w3578, "MulticolumnListbox Ref in"=w3574, "refnum"=w3579) -> ("error out"=w3576:errorcluster, "Refnum out"=w3577:T59)  [unwired: 5 in, 2 out]
                            n2179 = call <vilib>:"Close Config Data.vi"("error in (no error)"=w3576, "refnum"=w3577) -> ("error out"=w3567:errorcluster)  [unwired: 8 in, 1 out]
                            n2180 = Path To String(path=w3569) -> (string=w3570:string)
                            n2181 = local write "ini File Error"(w3567) -> ()
                            n2182 = Concatenate Strings(w3571, w3570, w3571, " saved. " ("string")) -> (w3568:string)
                          }
                          frame True {
                            # "Use DB"
                            n2183 = call "DB - [MasterData].[Procedure].vi"("DB - Master Data Enum"=DB_-_Master_Data_Procedure_Enum."INSERT [MasterData].[Procedure]", "MCListbox Refnum"=w3584, "Clust Refnum"=w3582) -> ("connection reference"=w3588:T66, "SUMMARY"=w3587:errorcluster)  [unwired: 9 in, 2 out]
                            n2184 = call "DB - [MasterData].[Procedure].vi"("connection reference"=w3588, "DB - Master Data Enum"=DB_-_Master_Data_Procedure_Enum."INSERT [MasterData][ProcedureItem]", "error in (no error)"=w3587, "MCListbox Refnum"=w3584, "Clust Refnum"=w3582) -> ("SUMMARY"=w3583:errorcluster)  [unwired: 7 in, 3 out]
                            "DB" <- w3583
                          }
                        }
                        n2185 = property class="Clust (strict)"(reference=w3560) -> ("Value"=w3559:T13)  [unwired: 1 in, 2 out]
                        n2186 = Unbundle By Name(w3559) -> ("Master Data WPS/Ref"=w3556:T5, "Master Data Rev"=w3555:T5)
                        n2187 = case shown="Error" w3561 {
                          tunnel: [" WPS details saved." ("string") " WPS Details cannot be saved." ("string")] -> w3564
                          tunnel: w3562 -> [_ _]
                          tunnel: ["<I 522>" ("<.?....> Message Code") "<E 525>" ("<.?....> Message Code")] -> w3558
                          tunnel: ["WPS Saved. " ("string") "WPS save Failed" ("string")] -> w3557
                          frame No Error {
                            # "File/DB Save OK"
                          }
                          frame Error {
                            # "File/DB Save Not OK"
                          }
                        }
                        n2188 = call "String - Create comma seperated String.vi"("B"=w3555, "A"=w3556) -> ("A, B , C (auto comma)"=w3554:string)  [unwired: 9 in]
                      }
                    }
                    n2189 = call "Msgbox - Message Handler.vi"("Short Description (When DB Not Available)"=w3538, "Description (When DB Not Available)"=w3541, "Pre-Description"=w3540, "<.?....> Message Code"=w3539) -> ("MHandler Error"=w3542:errorcluster)  [unwired: 5 in, 2 out]
                    n2190 = local write "MHandler"(w3542) -> ()
                  }
                  frame True {
                    w3608 = 0 ("index (row)")
                    # "Goto RC"
                    # "Highlight 1st row of empty fields"
                    # "Header Complete, FHS has Empty Cells - No Saving"
                    n2191 = Index Array(array=w3613, index (row) #1=w3608, index (col) #1=w3608, index (row) #2=w3608, index (col) #2=1 ("disabled index (col)")) -> (element #1=w3606:i32, element #2=w3605:i32)
                    n2192 = Bundle("Numeric Control"=w3606, "Numeric Control"=w3605) -> (w3604:T71)  [unwired: 1 in]
                    n2193 = property class="MCListbox (strict)"(reference=w3614, "Value"=w3606, "EditPos"=w3604) -> ()  [unwired: 1 in, 2 out]
                    n2194 = for {
                      tunnel: w3613 -> [w3624] mode=indexing
                      shift-right: [w3615] -> w3612
                      shift-left: "" -> [w3617]
                      n2195 = Increment(x=w3624) -> (x+1=w3623:i32[])
                      n2196 = Number To Decimal String(number=w3623) -> (decimal integer string=w3622:string[])  [unwired: 1 in]
                      n2197 = Index Array(array=w3622) -> (element #1=w3620:string, element #2=w3618:string)  [unwired: 2 in]
                      n2198 = Concatenate Strings(w3617, " R" ("string"), w3620, "C" ("string"), w3618, "," ("string")) -> (w3615:string)
                    }
                    n2199 = String Length(string=w3612) -> (length=w3610:i32)
                    n2200 = Decrement(x=w3610) -> (x-1=w3609:i32)
                    n2201 = Replace Substring(3:w3609, 4:"." ("substring (\"\")"), 5:w3612) -> (1:w3601:string)  [unwired: 1 in, 1 out]
                    n2202 = Select(t=w3601, s=w3603, f="Table " ("string")) -> (s? t:f=w3600:string)
